vi "Stop Core.vi"(10 "final error code":i32, 11 "Detector_panel in":refnum<class "Detector_panel.lvclass">) -> (3 "Detector_panel out":refnum<class "Detector_panel.lvclass">)   [LabVIEW 2015, in "Detector_panel.lvclass"]
doc: "(<B>Filename</B>: Actor Framework.lvlib:Actor.lvclass:Stop Core.vi)\n\nDefines what the actor does before it stops. Use the <B>final error code</B> input to determine whether the actor shut down in response to an error.\n\nBy default, this method does nothing. A descendant class may override it to define behavior, such as shutting down any processes the actor initiated in its override of the Actor Core method."
uses:
  Detector_panel.lvclass
  UI/panel_class/panel.lvclass
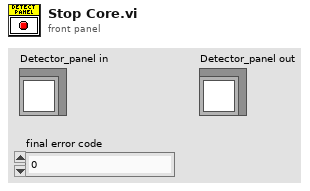
[diagram p1: front panel]
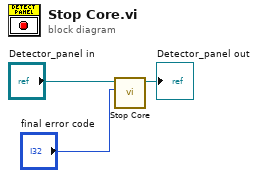
[diagram p0: block diagram]
diagram:
  n1 = call-parent "Stop Core.vi"("final error code"="final error code", "Actor in"="Detector_panel in") -> ("Actor out"=→"Detector_panel out":refnum<class "Detector_panel.lvclass">)  [unwired: 9 in]
